vi "CentreAnnulusROIonMatchPOS (SubVI).vi"(1 "Matches (pixel)":T1(array[cluster]), 2 "Annulus ROI Descriptor":T3={"Global Rectangle"=[675, 567, 1751, 1642], "Contours"=[{"ID"=enum."External", "Type"=7, "Coordinates"=[1212, 1104, 85, 537, 0, 0]}]} {"Contours"."Type" items=["No Selection", "Point", "Line", "Rectangle", "Oval", "Polygon", "Freehand Region", "Annulus", "Unused2", "Unused3", "Broken Line", "Freehand Line", "Rotated Rectangle"]}) -> (0 "Annulus ROI Descriptor centred on match position":T2)   [LabVIEW 2016]
panel:
  # "85"
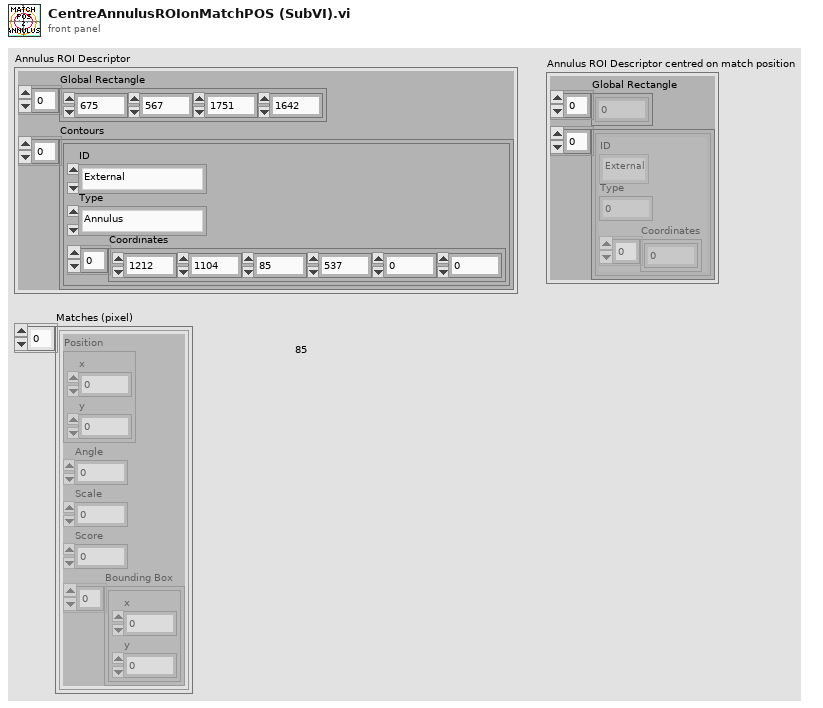
[diagram p1: front panel]
types:
  T1 = cluster{"Position":cluster{"x":sgl, "y":sgl}, "Angle":sgl, "Scale":sgl, "Score":sgl, "Bounding Box":cluster{"x":sgl, "y":sgl}[]}[]
  T2 = cluster{"Global Rectangle":i32[], cluster{"ID":enum32{"External", "Internal"}, "Type":u32, "Coordinates":i32[]}[]}
  T3 = cluster{"Global Rectangle":i32[], "Contours":cluster{"ID":enum32{"External", "Internal"}, "Type":u32, "Coordinates":i32[]}[]}
  T4 = cluster{"ID":enum32{"External", "Internal"}, "Type":u32, "Coordinates":i32[]}[]
  T5 = cluster{"ID":enum32{"External", "Internal"}, "Type":u32, "Coordinates":i32[]}
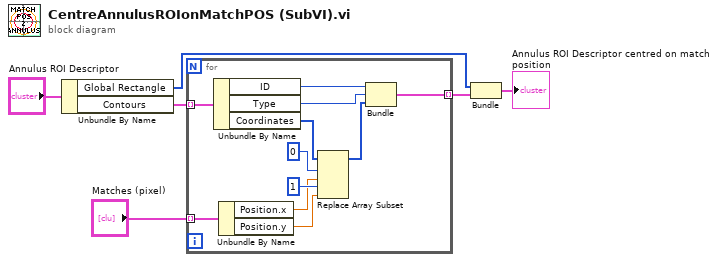
[diagram p0: block diagram]
diagram:
  n1 = Unbundle By Name("Annulus ROI Descriptor") -> ("Global Rectangle"=w4:i32[], "Contours"=w2:T4)
  n2 = for {
    tunnel: w2 -> [w17] mode=indexing
    tunnel: "Matches (pixel)" -> [w13] mode=indexing
    tunnel: [w7] -> w5 mode=indexing
    n3 = Unbundle By Name(w17) -> ("ID"=w8:enum32{"External", "Internal"}, "Type"=w10:u32, "Coordinates"=w16:i32[])
    n4 = Unbundle By Name(w13) -> ("Position.x"=w12:sgl, "Position.y"=w11:sgl)
    n5 = Replace Array Subset(array=w16, new element #1=w12, index #1=0 ("index"), new element #2=w11, index #2=1 ("index")) -> (w9:i32[])
    n6 = Bundle("ID"=w8, "Type"=w10, "Coordinates"=w9) -> (w7:T5)  [unwired: 1 in]
  }
  n7 = Bundle("Global Rectangle"=w4, w5) -> (→"Annulus ROI Descriptor centred on match position":T2)  [unwired: 1 in]
